vi "GetU32ImageArray.vi"(8 "error in (no error)":errorcluster) -> (0 "error out":errorcluster, 2 "OutputPixels":u32[](array[numeric]), 3 "Image Pixels":u32[][](array[numeric]), 4 "return":i32)   [LabVIEW 2015]
uses:
  [Global] Image.vi
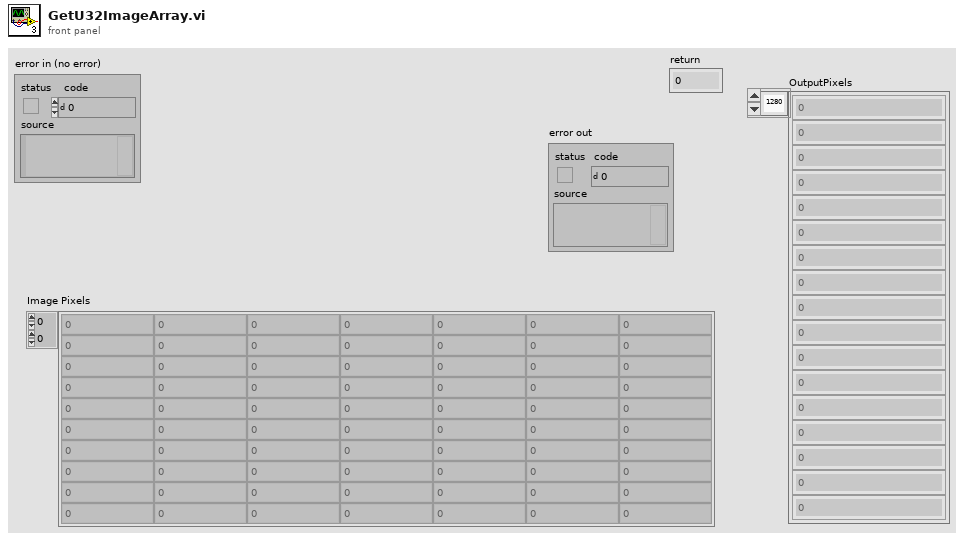
[diagram p1: front panel]
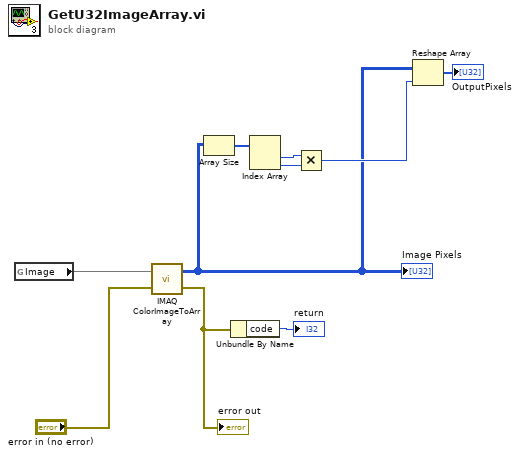
[diagram p0: block diagram]
diagram:
  n1 = global read "[Global] Image.vi" "Image"() -> (w9)
  n2 = call "IMAQ ColorImageToArray"("Image"=w9, "error in (no error)"="error in (no error)") -> ("Image Pixels (U32)"=w1:u32[][], "error out"=w7:errorcluster)  [unwired: 2 in, 1 out]
  "Image Pixels" <- w1
  "error out" <- w7
  n3 = Array Size(array=w1) -> (size(s)=w6:i32[])
  n4 = Unbundle By Name(w7) -> ("code"=→"return":i32)
  n5 = Index Array(array=w6) -> (element #1=w4:i32, element #2=w5:i32)  [unwired: 2 in]
  n6 = Multiply(x=w4, y=w5) -> (x*y=w3:i32)
  n7 = Reshape Array(w1, w3) -> (→"OutputPixels":u32[])
